vi "niRFUtil FTW Generate Flat Response.vi"(2 "Minimum Selectivity (dB)":dbl=70.0 format="%.2f", 3 "df (Hz)":dbl format="%^.2e", 4 "Bandwidth (Hz)":T3 format="%^.3e", 5 "Center Frequency (Hz)":dbl format="%^.2e") -> (0 "-ENBW (dB-Hz)":sgl format="%.2f", 1 "Filter Power Response":T1 {"y" min=0 max=127 format="%.2f"; "dx" format="%^.2e"; "x0" format="%^.2e"})   [LabVIEW 2015, in "niRFUtil.lvlib"]
doc: "(c) Copyright 2006, National Instruments, Inc. This VI may not be duplicated, sold, or distributed without written consent from National Instruments."
uses:
  niRFUtil.lvlib
  Includes/niRFUtil INC RBW Filter Bandwidth.ctl
  Includes/niRFUtil INC Real Waveform.ctl
  Includes/niRFUtil INC Real Array.ctl
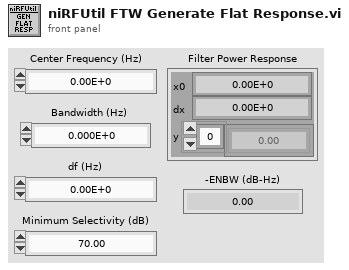
[diagram p1: front panel]
types:
  T1 = typedef "niRFUtil.lvlib/niRFUtil INC Real Waveform.ctl" = cluster{"x0":dbl, "dx":dbl, "y":T2}
  T2 = typedef "niRFUtil.lvlib/niRFUtil INC Real Array.ctl" = sgl[]
  T3 = typedef "niRFUtil.lvlib/niRFUtil INC RBW Filter Bandwidth.ctl" = dbl
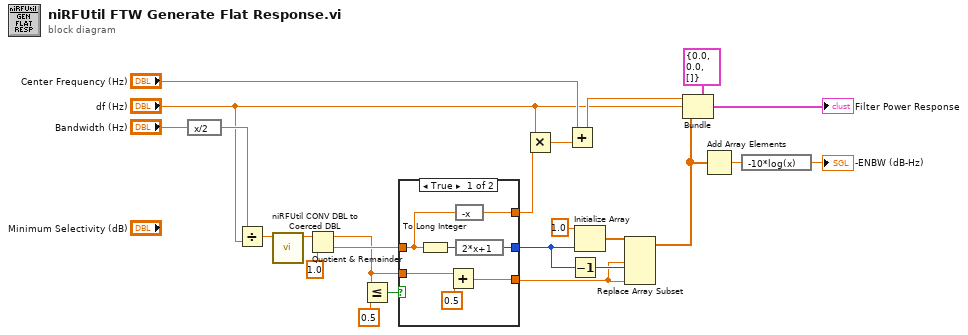
[diagram p0: block diagram]
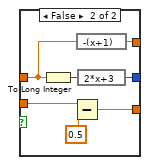
[diagram p2: hidden frame]
diagram:
  n1 = expression code="x/2"("Bandwidth (Hz)") -> (w20:T3)
  n2 = Divide(x=w20, y="df (Hz)") -> (x/y=w14:T3)
  n3 = call "niRFUtil CONV DBL to Coerced DBL.vi"("Numeric In (DBL)"=w14) -> ("Coerced Numeric Out (DBL)"=w23:dbl)  [unwired: 10 in]
  n4 = Quotient & Remainder(x=w23, y=1.0) -> (x-y*floor(x/y)=w8:dbl, floor(x/y)=w10:dbl)
  n5 = Less Or Equal?(x=w8, y=0.5) -> (x <= y?=w11:bool)
  n6 = case shown="True" w11 {
    tunnel: w10 -> [w26 w33]
    tunnel: [w30 w37] -> w9
    tunnel: w8 -> [w28 w35]
    tunnel: [w27 w34] -> w7
    tunnel: [w25 w32] -> w6
    frame True {
      n7 = To Long Integer(number=w26) -> (32bit integer=w31:i32)
      n8 = Add(x=w28, y=0.5) -> (x+y=w27:dbl)
      n9 = expression code="-x"(w26) -> (w25:dbl)
      n10 = expression code="2*x+1"(w31) -> (w30:i32)
    }
    frame False {
      n11 = To Long Integer(number=w33) -> (32bit integer=w38:i32)
      n12 = Subtract(x=w35, y=0.5) -> (x-y=w34:dbl)
      n13 = expression code="-(x+1)"(w33) -> (w32:dbl)
      n14 = expression code="2*x+3"(w38) -> (w37:i32)
    }
  }
  n15 = Multiply(x="df (Hz)", y=w6) -> (x*y=w18:dbl)
  n16 = Add(x="Center Frequency (Hz)", y=w18) -> (x+y=w19:dbl)
  n17 = Decrement(x=w9) -> (x-1=w13:i32)
  n18 = Initialize Array(sgl 1.0 ("element"), w9) -> (w22:sgl[])
  n19 = Replace Array Subset(array=w22, new element #1=w7, new element #2=w7, index #2=w13) -> (w24:sgl[])  [unwired: 1 in]
  n20 = Bundle(cluster=T1 {"x0"=0.0, "dx"=0.0, "y"=[]} ("Filter Power Response"), "x0"=w19, "dx"="df (Hz)", "y"=w24) -> (→"Filter Power Response":T1)
  n21 = Add Array Elements(numeric array=w24) -> (sum=w21:sgl)
  n22 = expression code="-10*log(x)"(w21) -> (→"-ENBW (dB-Hz)":sgl)
